vi "ReadWrite.Data.Write.vi"(8 "error in":errorcluster, 9 "Offset":i32, 10 "Values":dbl[](array[numeric]), 11 "Ref":T1) -> (0 "error out":errorcluster)   [LabVIEW 2027, in "Data Access Engine (Express).lvlib" / "Data Access Engine (Express).lvclass"]
uses:
  Data Access Engine (Express).lvclass
  Types/ReadWrite.DVR.ctl
  Access Type Classes/ReadWrite/ReadWrite.lvclass
  Access Type Classes/ReadWrite/ReadWrite.lvclass/ReadWrite.ctl
  Access Type Classes/ReadWrite/ReadWrite.ProcessData.Buffer.vi
  Access Type Classes/ReadWrite/ReadWrite.ProcessData.Commit.vi
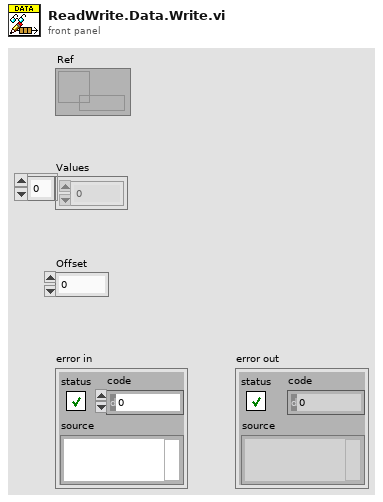
[diagram p1: front panel]
types:
  T1 = typedef "Data Access Engine (Express).lvlib/Data Access Engine (Express).lvclass/ReadWrite.DVR.ctl" = refnum<data-value>
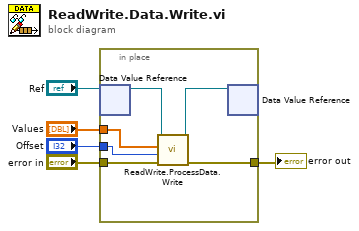
[diagram p0: block diagram]
diagram:
  n1 = in-place {
    in-place-border: "error in" -> [w9]
    in-place-border: [w8] -> w3
    in-place-border: "Values" -> [w7]
    in-place-border: "Offset" -> [w6]
    n2 = in-place-dvr #1("Ref") -> (w11:refnum<class "ReadWrite.lvclass">)  [unwired: 1 out]
    n3 = call "ReadWrite.ProcessData.Write.vi"("error in"=w9, "Offset"=w6, "Values"=w7, "ReadWrite in"=w11) -> ("error out"=w8:errorcluster, "ReadWrite out"=w10:refnum<class "ReadWrite.lvclass">)  [unwired: 5 in]
    n4 = in-place-dvr #1(w10) -> ()  [unwired: 2 out]
  }
  "error out" <- w3
